vi "Read MsgRX.vi"(8 "error in (no error)":errorcluster, 11 "Comm in":refnum<class "Comm.lvclass">) -> (0 "error out":errorcluster, 2 "MsgRX":string, 3 "Comm out":refnum<class "Comm.lvclass">)   [LabVIEW 2012, in "Comm.lvclass"]
uses:
  Comm.lvclass
  Comm.lvclass/Comm.ctl
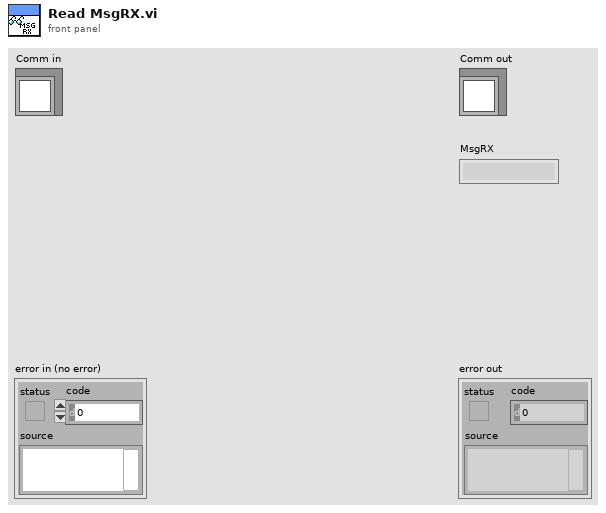
[diagram p1: front panel]
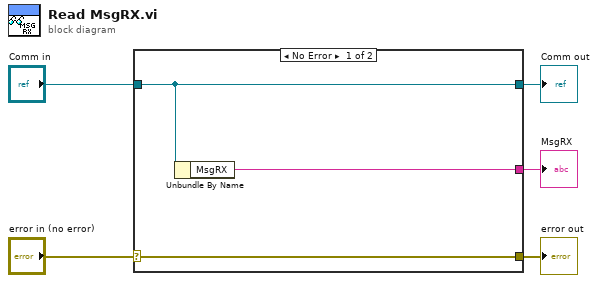
[diagram p0: block diagram]
diagram:
  n1 = case shown="No Error" "error in (no error)" {
    selector: "error in (no error)" -> [w8 w9]
    tunnel: [w8 w9] -> w4
    tunnel: [w7 w10] -> w2
    tunnel: "Comm in" -> [w7 w10]
    tunnel: [w6 _] -> w1
    frame No Error {
      n2 = Unbundle By Name(w7) -> ("MsgRX"=w6:string)
    }
    frame Error {
    }
  }
  "error out" <- w4
  "Comm out" <- w2
  "MsgRX" <- w1
